vi "Set Match Window.vi"(8 "error in (no error)":errorcluster, 10 "Match Time Window":dbl, 11 "Controller in":refnum<class "Controller.lvclass">) -> (0 "error out":errorcluster, 3 "Controller out":refnum<class "Controller.lvclass">)   [LabVIEW 2019, in "Controller.lvlib" / "Controller.lvclass"]
uses:
  Controller.lvclass
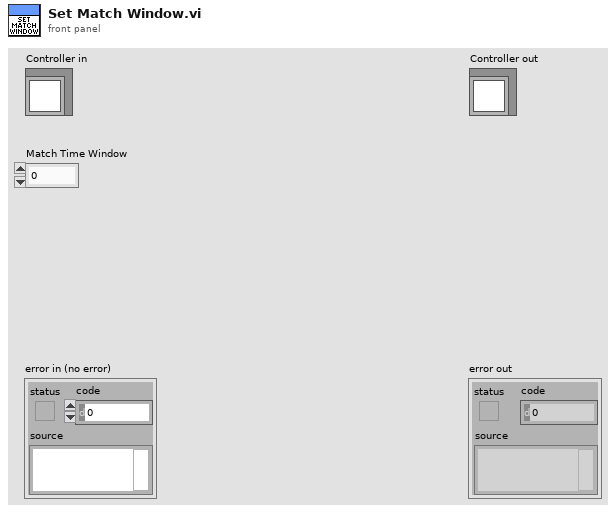
[diagram p1: front panel]
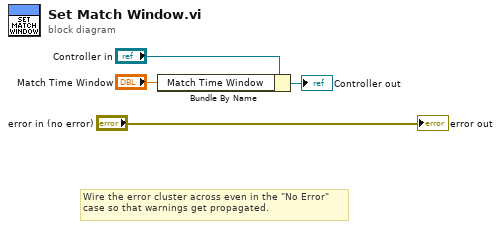
[diagram p0: block diagram]
diagram:
  # "Wire the error cluster across even in the \"No Error\"\ncase so that warnings get propagated."
  n1 = Bundle By Name(cluster="Controller in", "Match Time Window"="Match Time Window") -> (→"Controller out":refnum<class "Controller.lvclass">)
  "error out" <- "error in (no error)"
